vi "Global connessione strumenti.vi"() -> ()   [LabVIEW 2019]
panel:
  out "DCREG cpnnesso":bool
  out "Sinus penta connesso":bool
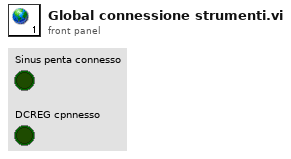
[diagram p1: front panel]
diagram:
